vi "ToTable.vi"(8 "error in":errorcluster, 9 "Table Index (0)":i32, 10 "variant":variant, 11 "JSON_RPC_Interface editor node in":refnum<class "JSON_RPC_Interface editor node.lvclass">) -> (0 "error out":errorcluster, 1 "row headers":string[](array[string]), 2 "table":string[][](array[string]), 3 "JSON_RPC_Interface editor node out":refnum<class "JSON_RPC_Interface editor node.lvclass">)   [LabVIEW 2018, in "JSON_RPC_Interface editor node.lvclass"]
doc: "Generates the strings needed to display on a table based on the information found in the engine and module configuration classes."
uses:
  JSON_RPC_Interface editor node.lvclass
  module/configuration/JSON_RPC_Interface configuration.lvclass
  C:/Program Files (x86)/National Instruments/LabVIEW 2018/vi.lib/NI/Configuration Framework/serializable configuration/NISE_CEF_serializable configuration.lvclass
  <vilib>/NI/Module Execution Interface/Engine Configuration/engine configuration.lvclass
  module/configuration/JSON_RPC_Interface configuration.lvclass/JSON_RPC_Interface configuration.ctl
  <vilib>/NI/Configuration Framework/serializable configuration/NISE_CEF_serializable configuration.lvclass/NISE_CEF_serializable configuration.ctl
  <vilib>/NI/Tag Bus Module Framework/channel/TBM channel.lvclass/TBM channel.ctl
  <vilib>/NI/Tag Bus/tag/tag descriptor.lvclass/tag descriptor.ctl
  module/configuration/Read Lines.vi
  <vilib>/NI/Tag Bus Module Framework/channel/TBM channel.lvclass
  C:/Program Files (x86)/National Instruments/LabVIEW 2018/vi.lib/NI/Tag Bus/tag/tag descriptor.lvclass
  <vilib>/Utility/LVClass/Get LV Class Name.vi
  <vilib>/NI/Configuration Framework/error generator/NISE_error generator.vi
  <vilib>/NI/Tag Bus/tag/tag descriptor.lvclass
  <vilib>/NI/Configuration Framework/serializable configuration/NISE_CEF_serializable configuration.lvclass
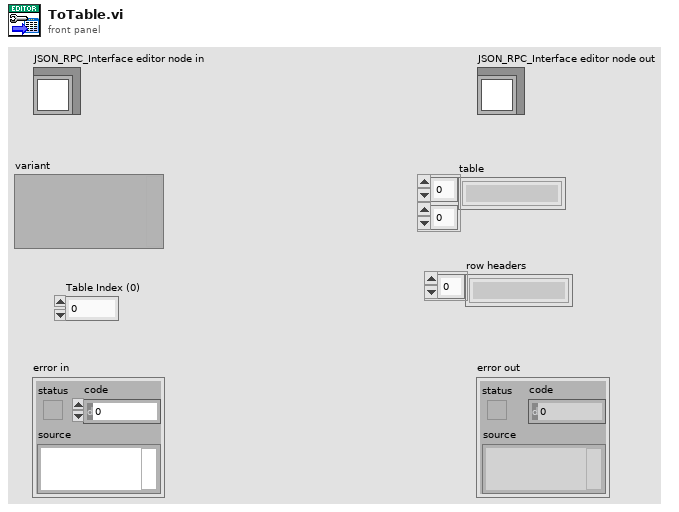
[diagram p1: front panel]
types:
  T1 = typedef "tag bus configurable plugin module configuration.lvclass/Line.ctl" = cluster{"channel":refnum<class "TBM channel.lvclass">}
  T2 = typedef "TBM channel.lvclass/channel classification.ctl" = enum16{"input data", "output data", "processing parameter", "processing result"}
  T3 = typedef "tag bus.lvlib/tag descriptor.lvclass/Data Type.ctl" = enum16{"Double", "Single", "I64", "I32", "I16", "I8", "U64", "U32", "U16", "U8", "Boolean", "String", "Array of Double", "Array of Single", "Array of I64", "Array of I32", "Array of I16", "Array of I8", "Array of U64", "Array of U32", "Array of U16", "Array of U8", "Array of Boolean", "Array of String"}
  T4 = typedef "JSON_RPC_Interface editor node.lvclass/permissions.ctl" = enum32{"Read from Engine", "Write to Engine"}
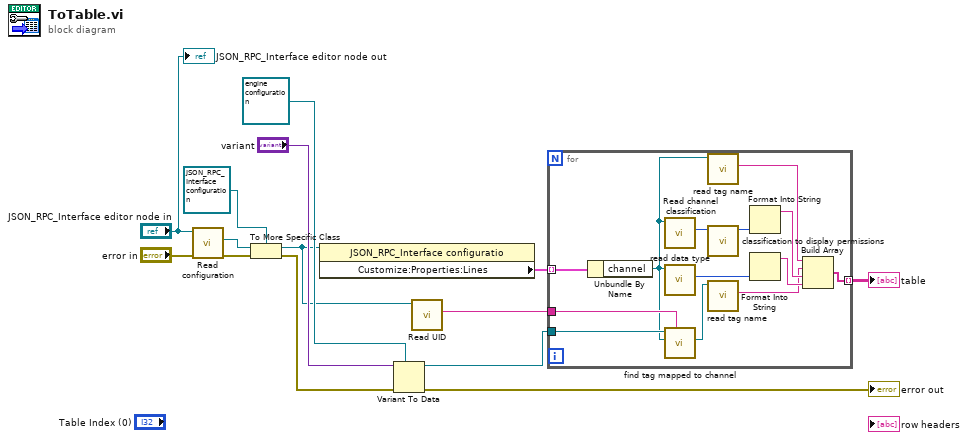
[diagram p0: block diagram]
diagram:
  n1 = call-dynamic "Read configuration.vi"("error in"="error in", "JSON_RPC_Interface editor node in"="JSON_RPC_Interface editor node in") -> ("error out"=w14:errorcluster, "configuration"=w5:refnum<class "NISE_CEF_serializable configuration.lvclass">)  [unwired: 7 in, 1 out]
  n2 = To More Specific Class(target class=refnum<class "JSON_RPC_Interface configuration.lvclass"> refnum ("tag bus configurable plugin module configuration"), reference=w5, error in=w14) -> (specific class reference=w4:refnum<class "JSON_RPC_Interface configuration.lvclass">, error out=w2:errorcluster)
  n3 = property class="JSON_RPC_Interface configuratio"(reference=w4) -> ("Customize:Properties:Lines"=w11:T1[])  [unwired: 1 in, 2 out]
  n4 = Variant To Data(error in=w2, type=refnum<class "engine configuration.lvclass"> refnum ("engine configuration"), Variant="variant") -> (data=w8:refnum<class "engine configuration.lvclass">, error out=→"error out":errorcluster)
  n5 = call <vilib>:"Read UID.vi"("configuration in"=w4) -> ("instance id"=w3:string)  [unwired: 8 in, 2 out]
  n6 = for {
    tunnel: w11 -> [w27] mode=indexing
    tunnel: w8 -> [w26]
    tunnel: [w19] -> w6 mode=indexing
    tunnel: w3 -> [w18]
    n7 = Unbundle By Name(w27) -> ("channel"=w16:refnum<class "TBM channel.lvclass">)
    n8 = call <vilib>:"Read channel classification.vi"("channel in"=w16) -> ("channel classification"=w24:T2)  [unwired: 8 in, 2 out]
    n9 = call <vilib>:"read data type.vi"("system tag in"=w16) -> ("data type"=w21:T3)  [unwired: 8 in, 2 out]
    n10 = call <vilib>:"find tag mapped to channel.vi"("owner"=w18, "channel"=w16, "engine configuration in"=w26) -> ("tag"=w25:refnum<class "tag descriptor.lvclass">)  [unwired: 6 in, 2 out]
    n11 = call <vilib>:"read tag name.vi"("system tag in"=w16) -> ("name"=w15:string)  [unwired: 8 in, 2 out]
    n12 = call "classification to display permissions.vi"("channel classification"=w24) -> ("permissions"=w23:T4)  [unwired: 10 in]
    n13 = call <vilib>:"read tag name.vi"("system tag in"=w25) -> ("name"=w17:string)  [unwired: 8 in, 2 out]
    n14 = Format Into String(w23) -> (resulting string=w22:string)  [unwired: 3 in, 1 out]
    n15 = Format Into String(w21) -> (resulting string=w20:string)  [unwired: 3 in, 1 out]
    n16 = Build Array(w15, w17, w22, w20) -> (w19:string[])
  }
  "table" <- w6
  "JSON_RPC_Interface editor node out" <- "JSON_RPC_Interface editor node in"
